vi "Get station global.vi"(8 "error in (no error)":errorcluster, 11 "Global name":string="test_pc_name") -> (0 "error out":errorcluster, 1 "no?":bool, 2 "yes?":bool, 3 "Global value":string)   [LabVIEW 2013]
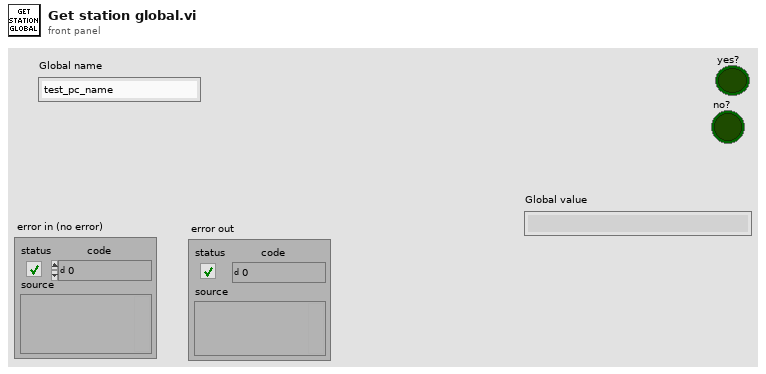
[diagram p1: front panel]
types:
  T1 = cluster{"Test folder":string, "Top level":string, "Main":string, "Test report":string, "Work order qty":string, "Work order meid":string, "Work order imei":string, "Master meid imei list":string, "Master test data":string, "ZPL label info":string, "Pictures":string, "Setup info":string, "Work order":string, "Tests folder":string, "Tests steps folder":string, "Config folder":string, "Verizon Upload file":string, "Job data file":string, "Station globals":string, "Post test info":string}
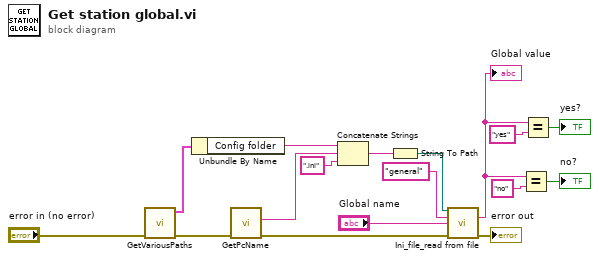
[diagram p0: block diagram]
diagram:
  n1 = call "GetVariousPaths.vi"("error in (no error)"="error in (no error)") -> ("error out"=w15:errorcluster, "Built Paths"=w16:T1)  [unwired: 9 in]
  n2 = Unbundle By Name(w16) -> ("Config folder"=w4:string)
  n3 = call "GetPcName.vi"("error in (no error)"=w15) -> ("error out"=w12:errorcluster, "Basic Name"=w14:string)  [unwired: 7 in, 2 out]
  n4 = Concatenate Strings(w4, w14, ".ini" ("string")) -> (w3:string)
  n5 = String To Path(string=w3) -> (path=w2:path)
  n6 = call "Ini_file_read from file.vi"("config file path"=w2, "Section Name"="general", "Key Name"="Global name", "error in (no error)"=w12) -> ("Key data from file"=w1:string, "error out"=→"error out":errorcluster)  [unwired: 8 in, 2 out]
  "Global value" <- w1
  n7 = Equal?(x=w1, y="no") -> (x = y?=→"no?":bool)
  n8 = Equal?(x=w1, y="yes") -> (x = y?=→"yes?":bool)
